vi "Manual Generation of WiBCI16T Channel Settings.vi"(8 "error in (no error)":errorcluster) -> (0 "error out":errorcluster)   [LabVIEW 2016, in "Settings Editor.lvlib"]
doc: "Get the path to the Settings XML file. This is done using the Application Directory function. For more information on how Application Directory calculates its path, right-click the function and choose Help.\n_____\nBased on DQMH Project Template 6.1.0.94."
uses:
  Settings Editor.lvlib
  CML Shared/EEG Channel Settings.ctl
  CML Shared/CML Shared.lvlib
  <vilib>/Utility/xml.llb/Write to XML File(string).vi
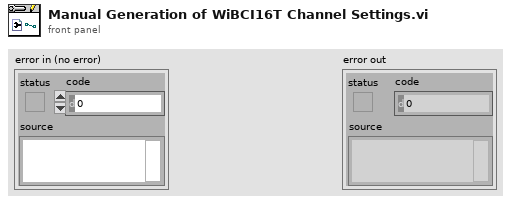
[diagram p1: front panel]
types:
  T1 = typedef "CML Shared.lvlib/EEG Channel Settings.ctl" = cluster{"16 EEG Channels":cluster{"Channel Name":string, "Channel No":u8, "Channel Enabled":bool, "Channel Referenced":bool}[], "Gain":u8}
  T2 = cluster{"Channel Name":string, "Channel No":u8, "Channel Enabled":bool, "Channel Referenced":bool}[]
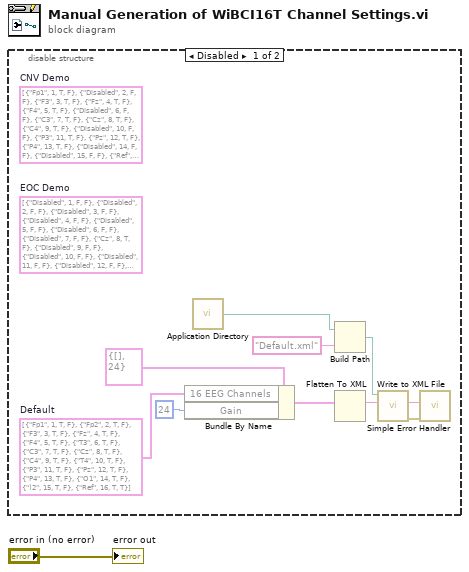
[diagram p0: block diagram]
diagram:
  n1 = disable-structure shown="Disabled" {
    frame Disabled {
      (unwired) T2 [{"Channel Name"="Fp1", "Channel No"=1, "Channel Enabled"=TRUE, "Channel Referenced"=FALSE}, {"Channel Name"="Disabled", "Channel No"=2, "Channel Enabled"=FALSE, "Channel Referenced"=FALSE}, {"Channel Name"="F3", "Channel No"=3, "Channel Enabled"=TRUE, "Channel Referenced"=FALSE}, {"Channel Name"="Fz", "Channel No"=4, "Channel Enabled"=TRUE, "Channel Referenced"=FALSE}, {"Channel Name"="F4", "Channel No"=5, "Channel Enabled"=TRUE, "Channel Referenced"=FALSE}, {"Channel Name"="Disabled", "Channel No"=6, "Channel Enabled"=FALSE, "Channel Referenced"=FALSE}, {"Channel Name"="C3", "Channel No"=7, "Channel Enabled"=TRUE, "Channel Referenced"=FALSE}, {"Channel Name"="Cz", "Channel No"=8, "Channel Enabled"=TRUE, "Channel Referenced"=FALSE}, {"Channel Name"="C4", "Channel No"=9, "Channel Enabled"=TRUE, "Channel Referenced"=FALSE}, {"Channel Name"="Disabled", "Channel No"=10, "Channel Enabled"=FALSE, "Channel Referenced"=FALSE}, {"Channel Name"="P3", "Channel No"=11, "Channel Enabled"=TRUE, "Channel Referenced"=FALSE}, {"Channel Name"="Pz", "Channel No"=12, "Channel Enabled"=TRUE, "Channel Referenced"=FALSE}, {"Channel Name"="P4", "Channel No"=13, "Channel Enabled"=TRUE, "Channel Referenced"=FALSE}, {"Channel Name"="Disabled", "Channel No"=14, "Channel Enabled"=FALSE, "Channel Referenced"=FALSE}, {"Channel Name"="Disabled", "Channel No"=15, "Channel Enabled"=FALSE, "Channel Referenced"=FALSE}, {"Channel Name"="Ref", "Channel No"=16, "Channel Enabled"=TRUE, "Channel Referenced"=TRUE}]  # CNV Demo
      w2 = T2 [{"Channel Name"="Fp1", "Channel No"=1, "Channel Enabled"=TRUE, "Channel Referenced"=FALSE}, {"Channel Name"="Fp2", "Channel No"=2, "Channel Enabled"=TRUE, "Channel Referenced"=FALSE}, {"Channel Name"="F3", "Channel No"=3, "Channel Enabled"=TRUE, "Channel Referenced"=FALSE}, {"Channel Name"="Fz", "Channel No"=4, "Channel Enabled"=TRUE, "Channel Referenced"=FALSE}, {"Channel Name"="F4", "Channel No"=5, "Channel Enabled"=TRUE, "Channel Referenced"=FALSE}, {"Channel Name"="T3", "Channel No"=6, "Channel Enabled"=TRUE, "Channel Referenced"=FALSE}, {"Channel Name"="C3", "Channel No"=7, "Channel Enabled"=TRUE, "Channel Referenced"=FALSE}, {"Channel Name"="Cz", "Channel No"=8, "Channel Enabled"=TRUE, "Channel Referenced"=FALSE}, {"Channel Name"="C4", "Channel No"=9, "Channel Enabled"=TRUE, "Channel Referenced"=FALSE}, {"Channel Name"="T4", "Channel No"=10, "Channel Enabled"=TRUE, "Channel Referenced"=FALSE}, {"Channel Name"="P3", "Channel No"=11, "Channel Enabled"=TRUE, "Channel Referenced"=FALSE}, {"Channel Name"="Pz", "Channel No"=12, "Channel Enabled"=TRUE, "Channel Referenced"=FALSE}, {"Channel Name"="P4", "Channel No"=13, "Channel Enabled"=TRUE, "Channel Referenced"=FALSE}, {"Channel Name"="O1", "Channel No"=14, "Channel Enabled"=TRUE, "Channel Referenced"=FALSE}, {"Channel Name"=")2", "Channel No"=15, "Channel Enabled"=TRUE, "Channel Referenced"=FALSE}, {"Channel Name"="Ref", "Channel No"=16, "Channel Enabled"=TRUE, "Channel Referenced"=TRUE}]  # Default
      (unwired) T2 [{"Channel Name"="Disabled", "Channel No"=1, "Channel Enabled"=FALSE, "Channel Referenced"=FALSE}, {"Channel Name"="Disabled", "Channel No"=2, "Channel Enabled"=FALSE, "Channel Referenced"=FALSE}, {"Channel Name"="Disabled", "Channel No"=3, "Channel Enabled"=FALSE, "Channel Referenced"=FALSE}, {"Channel Name"="Disabled", "Channel No"=4, "Channel Enabled"=FALSE, "Channel Referenced"=FALSE}, {"Channel Name"="Disabled", "Channel No"=5, "Channel Enabled"=FALSE, "Channel Referenced"=FALSE}, {"Channel Name"="Disabled", "Channel No"=6, "Channel Enabled"=FALSE, "Channel Referenced"=FALSE}, {"Channel Name"="Disabled", "Channel No"=7, "Channel Enabled"=FALSE, "Channel Referenced"=FALSE}, {"Channel Name"="Cz", "Channel No"=8, "Channel Enabled"=TRUE, "Channel Referenced"=FALSE}, {"Channel Name"="Disabled", "Channel No"=9, "Channel Enabled"=FALSE, "Channel Referenced"=FALSE}, {"Channel Name"="Disabled", "Channel No"=10, "Channel Enabled"=FALSE, "Channel Referenced"=FALSE}, {"Channel Name"="Disabled", "Channel No"=11, "Channel Enabled"=FALSE, "Channel Referenced"=FALSE}, {"Channel Name"="Disabled", "Channel No"=12, "Channel Enabled"=FALSE, "Channel Referenced"=FALSE}, {"Channel Name"="Disabled", "Channel No"=13, "Channel Enabled"=FALSE, "Channel Referenced"=FALSE}, {"Channel Name"="Disabled", "Channel No"=14, "Channel Enabled"=FALSE, "Channel Referenced"=FALSE}, {"Channel Name"="Disabled", "Channel No"=15, "Channel Enabled"=FALSE, "Channel Referenced"=FALSE}, {"Channel Name"="Ref", "Channel No"=16, "Channel Enabled"=TRUE, "Channel Referenced"=TRUE}]  # EOC Demo
      n2 = Bundle By Name(cluster=T1 {"16 EEG Channels"=[], "Gain"=24} ("EEG Channels"), "16 EEG Channels"=w2, "Gain"=u8 24 ("EEG Channels.Gain")) -> (w10:T1)
      n3 = call <vilib>:"Application Directory.vi"() -> ("Application Directory"=w3:path)
      n4 = Build Path(base path=w3, name or relative path="Default.xml") -> (appended path=w7:path)
      n5 = Flatten To XML(anything=w10) -> (xml string=w9:string)
      n6 = call-poly <vilib>:"Write to XML File.vi"("XML Input"=w9, "XML File Path"=w7) -> ("error out"=w5:errorcluster, "XML String"=w6:string)  [unwired: 7 in, 1 out]
      n7 = call <vilib>:"Simple Error Handler.vi"("error source (\" \")"=w6, "error in (no error)"=w5) -> ()  [unwired: 3 in, 5 out]
    }
    frame Enabled {
    }
  }
  "error out" <- "error in (no error)"
